vi "ColorText Facade.vi"(0 "Data In":T4, 2 "Display State In":T2, 3 "Container State":T3) -> (6 "Data Out":T4, 7 "Display State Out":T2, 8 "Action":T1)   [LabVIEW 2016, in "Code.xctl"]
uses:
  Code.xctl
  <vilib>/_xctls/Action.ctl
  <vilib>/_xctls/XControlSupport.lvlib
  <vilib>/_xctls/Container State.ctl
  ColorText Data.ctl
  ColorText State.ctl
panel:
  in  "Code":string
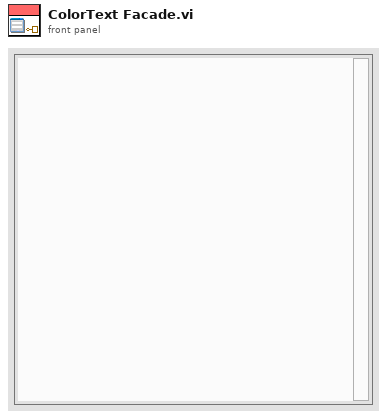
[diagram p1: front panel]
types:
  T1 = typedef "XControlSupport.lvlib/Action.ctl" = cluster{"Data Changed?":bool, "State Changed?":bool, "Action Name":string}
  T2 = typedef "Code.xctl/ColorText State.ctl" = cluster{"Numeric":dbl}
  T3 = typedef "XControlSupport.lvlib/Container State.ctl" = cluster{"Indicator?":bool, "Run Mode?":bool, " Refnum":refnum<vi>}
  T4 = typedef "Code.xctl/ColorText Data.ctl" = string
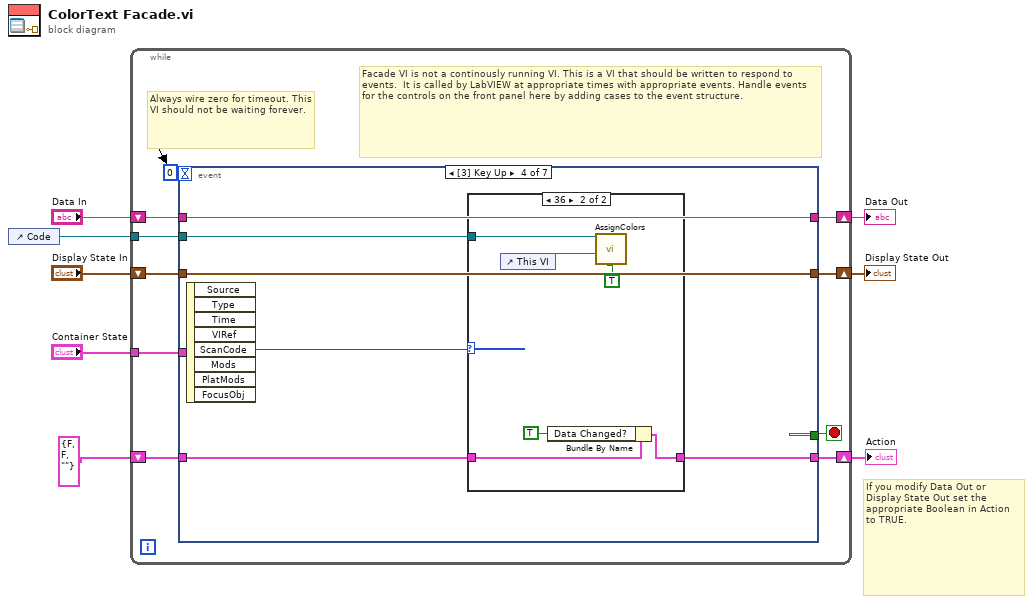
[diagram p0: block diagram]
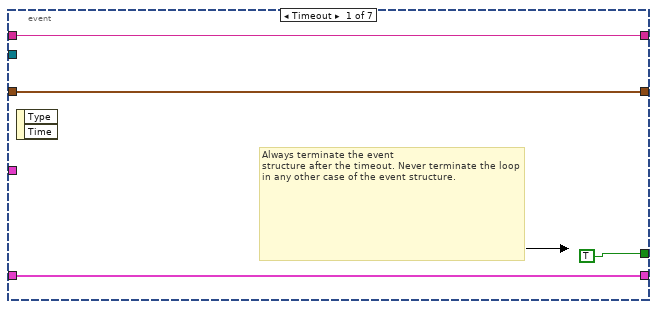
[diagram p2: hidden frame]
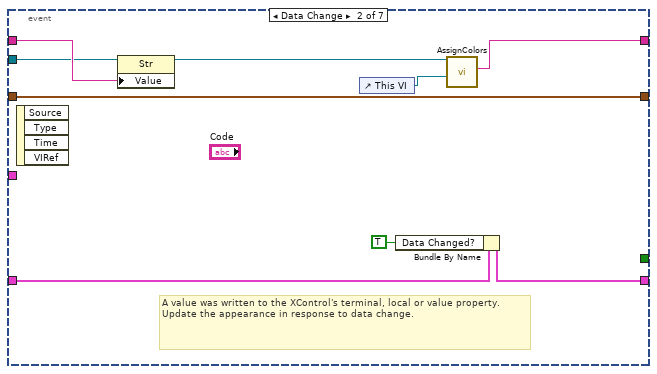
[diagram p3: hidden frame]
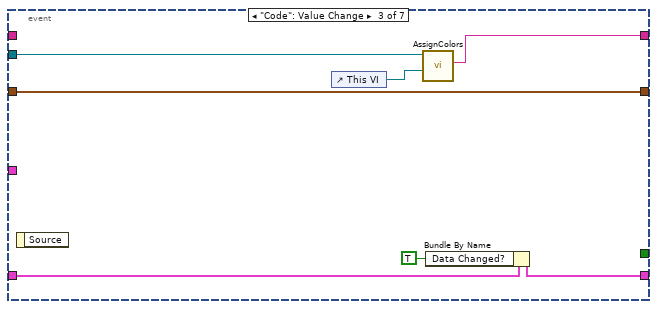
[diagram p4: hidden frame]
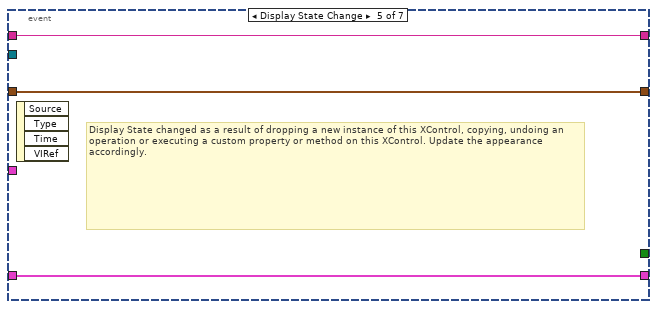
[diagram p6: hidden frame]
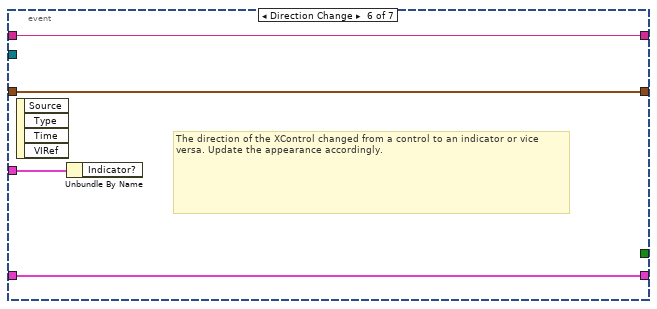
[diagram p7: hidden frame]
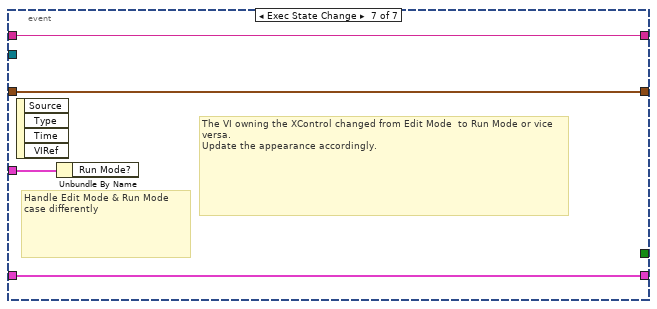
[diagram p8: hidden frame]
diagram:
  # "If you modify Data Out or\nDisplay State Out set the\nappropriate Boolean in Action\nto TRUE."
  n1 = control-ref of="Code"() -> (w1:refnum<vi>)
  n2 = while {
    shift-right: [w17] -> w5
    shift-left: "Display State In" -> [w18]
    tunnel: "Container State" -> [w14]
    shift-right: [w12] -> w8
    shift-left: "Data In" -> [w13]
    shift-right: [w10] -> w3
    shift-left: T1 {"Data Changed?"=FALSE, "State Changed?"=FALSE, "Action Name"=""} ("Action") -> [w11]
    tunnel: w1 -> [w9]
    stop <- w16 stop-if-true
    # "Facade VI is not a continously running VI. This is a VI that should be written to respond to events.  It is called by LabVIEW at appropriate times with appropriate events. Handle events for the controls on the front panel here by adding cases to the event structure."
    # "Always wire zero for timeout. This\nVI should not be waiting forever."
    n3 = event shown="[3] Key Up" {
      selector: _ -> [_ _ _ _ _ _ _]
      dyn-events: _ -> [_ _ _ _ _ _ _]
      timeout: 0 -> [_ _ _ _ _ _ _]
      tunnel: w18 -> [w20 w31 w38 w44 w54 w57 w61]
      tunnel: [w20 w31 w38 w44 w54 w57 w61] -> w17
      tunnel: [TRUE _ _ _ _ _ _] -> w16
      tunnel: w14 -> [_ _ _ _ _ w58 w62]
      tunnel: w13 -> [w19 w25 _ w43 w53 w56 w60]
      tunnel: [w19 w27 w34 w43 w53 w56 w60] -> w12
      tunnel: [w21 w29 w36 w39 w52 w55 w59] -> w10
      tunnel: w11 -> [w21 w30 w37 w40 w52 w55 w59]
      tunnel: w9 -> [_ w24 w33 w42 _ _ _]
      event Timeout {
        # "Always terminate the event\nstructure after the timeout. Never terminate the loop in any other case of the event structure."
        n4 = event-data() -> ()  [unwired: 1 in, 2 out]
      }
      event Data Change {
        # "A value was written to the XControl's terminal, local or value property.\nUpdate the appearance in response to data change."
        n5 = event-data() -> ()  [unwired: 1 in, 4 out]
        n6 = property on="Property Node" class="Str"(reference=w24, "Value"=w25) -> (reference out=w23:refnum<vi>)  [unwired: 1 in, 1 out]
        n7 = control-ref of="This VI"() -> (w26:refnum<vi>)
        n8 = Bundle By Name(cluster=w30, "Data Changed?"=TRUE) -> (w29:T1)
        n9 = call "AssignColors.vi"("Parent"=w26, "Code"=w23) -> ("Value"=w27:string)  [unwired: 9 in]
      }
      event "Code": Value Change {
        n10 = event-data() -> ()  [unwired: 1 in, 1 out]
        n11 = control-ref of="This VI"() -> (w32:refnum<vi>)
        n12 = call "AssignColors.vi"("Parent"=w32, "Code"=w33) -> ("Value"=w34:string)  [unwired: 9 in]
        n13 = Bundle By Name(cluster=w37, "Data Changed?"=TRUE) -> (w36:T1)
      }
      event Key Up {
        n14 = event-data() -> ("ScanCode"=w41:i16)  [unwired: 1 in, 7 out]
        n15 = case shown="36" w41 {
          tunnel: w42 -> [_ w50]
          tunnel: w40 -> [w45 w47]
          tunnel: [w45 w46] -> w39
          frame Default {
          }
          frame 36 {
            n16 = control-ref of="This VI"() -> (w49:refnum<vi>)
            n17 = Bundle By Name(cluster=w47, "Data Changed?"=TRUE) -> (w46:T1)
            n18 = call "AssignColors.vi"("Add Spaces?"=TRUE, "Parent"=w49, "Code"=w50) -> ()  [unwired: 8 in, 1 out]
          }
        }
      }
      event Display State Change {
        # "Display State changed as a result of dropping a new instance of this XControl, copying, undoing an operation or executing a custom property or method on this XControl. Update the appearance accordingly."
        n19 = event-data() -> ()  [unwired: 1 in, 4 out]
      }
      event Direction Change {
        # "The direction of the XControl changed from a control to an indicator or vice versa. Update the appearance accordingly."
        n20 = event-data() -> ()  [unwired: 1 in, 4 out]
        n21 = Unbundle By Name(w58) -> ()  [unwired: 1 out]
      }
      event Exec State Change {
        # "The VI owning the XControl changed from Edit Mode  to Run Mode or vice versa.\nUpdate the appearance accordingly."
        # "Handle Edit Mode & Run Mode\ncase differently"
        n22 = event-data() -> ()  [unwired: 1 in, 4 out]
        n23 = Unbundle By Name(w62) -> ()  [unwired: 1 out]
      }
    }
  }
  "Display State Out" <- w5
  "Data Out" <- w8
  "Action" <- w3
